vi "Create Arbitrary Waveform.vi"(7 "Arbitrary Waveform Name (0: USER1)":u16(ring) items=["USER1", "USER2", "USER3", "USER4"], 8 "error in (no error)":errorcluster, 9 "Arbitrary Waveform Data":dbl[](array[numeric]), 11 "VISA resource name":refnum<visa-resource-name>) -> (0 "error out":errorcluster, 3 "VISA resource name out":refnum<visa-resource-name>)   [LabVIEW 2019, in "Tektronix AFG 3000 Series.lvlib"]
doc: "Creates and saves an arbitrary waveform in edit memory. \n\n<B>Note:</B>\n\nCreates an arbitrary waveform in edit memory and because of this, the waveform will remain stored on the instrument until deleted. If any sensitive information is contained in the arbitrary waveform, it is recommended that the waveform be deleted when finished."
uses:
  <userlib>/Tektronix AFG 3000 Series/Tektronix AFG 3000 Series.lvlib
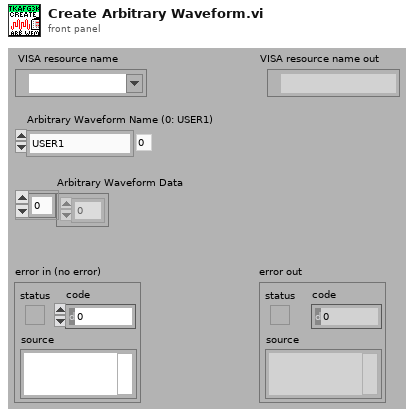
[diagram p1: front panel]
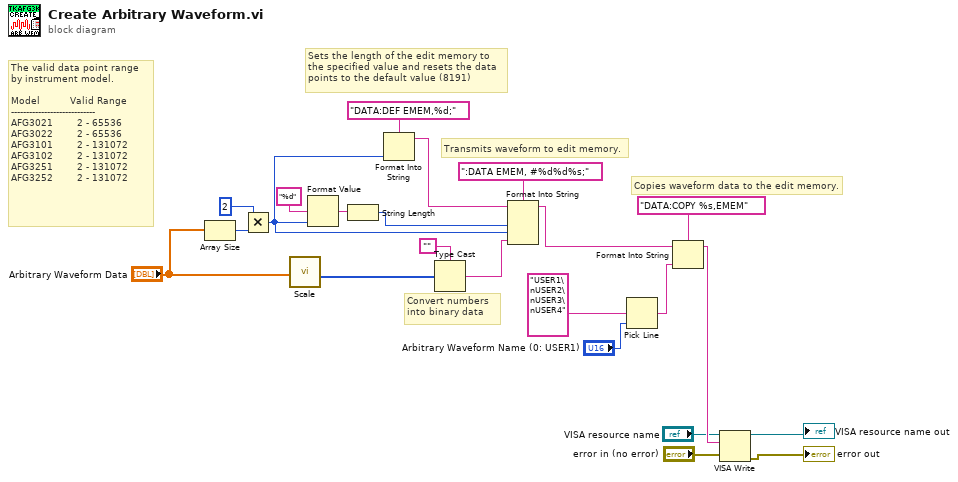
[diagram p0: block diagram]
diagram:
  # "The valid data point range \nby instrument model. \n\nModel          Valid Range\n----------------------------\nAFG3021        2 - 65536\nAFG3022        2 - 65536\nAFG3101        2 - 131072\nAFG3102        2 - 131072\nAFG3251        2 - 131072\nAFG3252        2 - 131072"
  # "Convert numbers\ninto binary data"
  # "Transmits waveform to edit memory."
  # "Sets the length of the edit memory to the specified value and resets the data points to the default value (8191)"
  # "Copies waveform data to the edit memory."
  n1 = Array Size(array="Arbitrary Waveform Data") -> (size(s)=w20:i32)
  n2 = Multiply(x=2, y=w20) -> (x*y=w7:i32)
  n3 = call <userlib>:"Scale.vi"("Waveform Data"="Arbitrary Waveform Data") -> ("Scaled Waveform Data"=w5:u16[])  [unwired: 10 in]
  n4 = Format Value(format string="%d", value (0)=w7) -> (output string=w10:string)  [unwired: 1 in]
  n5 = String Length(string=w10) -> (length=w9:i32)
  n6 = Format Into String(format string="DATA:DEF EMEM,%d;", w7) -> (resulting string=w13:string)  [unwired: 2 in, 1 out]
  n7 = Type Cast(type="", x=w5) -> (*(type *) &x=w12:string)
  n8 = Format Into String(format string=":DATA EMEM, #%d%d%s;", initial string=w13, w9, w7, w12) -> (resulting string=w8:string)  [unwired: 1 in, 1 out]
  n9 = Pick Line(multi-line string="USER1\nUSER2\nUSER3\nUSER4", line index="Arbitrary Waveform Name (0: USER1)") -> (output string=w16:string)  [unwired: 1 in]
  n10 = Format Into String(format string="DATA:COPY %s,EMEM", initial string=w8, w16) -> (resulting string=w15:string)  [unwired: 1 in, 1 out]
  n11 = VISA Write(VISA resource name="VISA resource name", write buffer=w15, error in (no error)="error in (no error)") -> (VISA resource name out=→"VISA resource name out":refnum<visa-resource-name>, error out=→"error out":errorcluster)  [unwired: 1 out]
